vi "S30c_dll F101.vi"() -> ()   [LabVIEW 2014, in "K_S30c_dll.lvlib"]
uses:
  K_S30c_dll.lvlib
  s30c.dll
panel:
  in  "Parameter 0 .. 5":u8[](array[numeric])
  out "Org. Parameter 0 .. 4":u8[](array[numeric])
  in  "Index":u8
  out "error out":errorcluster
  in  "error in":errorcluster
  in  "Dev Addr":u8=250
  # "Function101: Write a single configurtion byte, using funtion 100\n\nWarning!\n\nPlease be careful, using this function! \nWrong configuration changes the function of the device! \nMake sure that you save first the origignal configuration with function 100.\nIf your device supports F32 (5.20-4.1 and earlier), then use F33 instead of this function.\n\nusing s30c.dll\nKeller AG für Druckmesstechnik, 29.5.08 b.v."
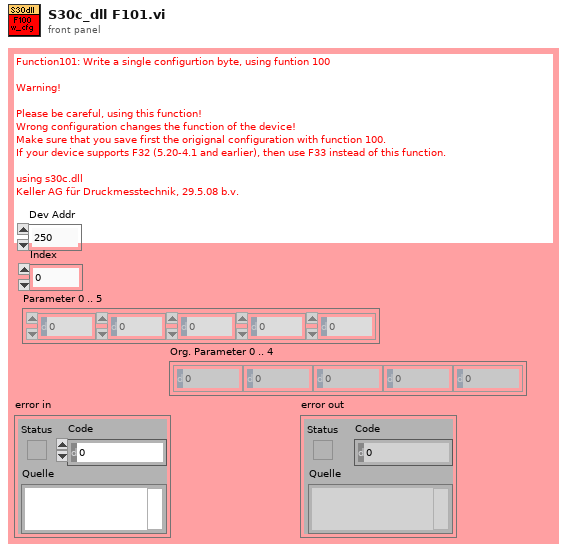
[diagram p1: front panel]
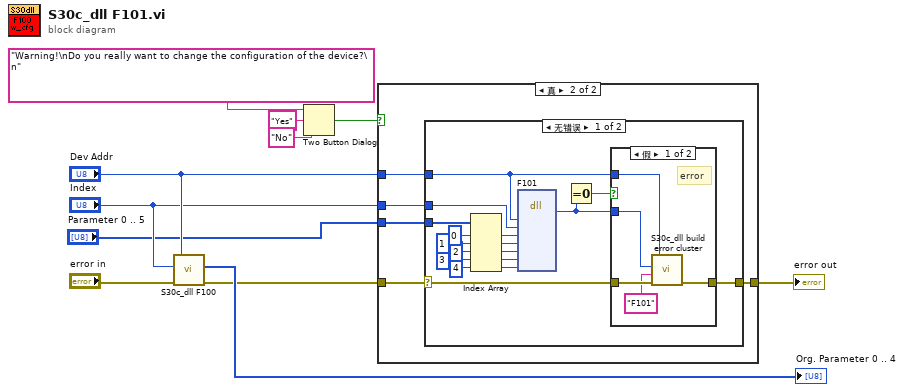
[diagram p0: block diagram]
diagram:
  n1 = call "S30c_dll F100.vi"("error in"="error in", "Index"="Index", "Dev Addr"="Dev Addr") -> ("error out"=w4:errorcluster, "Parameters 0 .. 4"=→"Org. Parameter 0 .. 4":u8[])  [unwired: 2 in, 1 out]
  n2 = Two Button Dialog(message="Warning!\nDo you really want to change the configuration of the device?\n" ("Nachricht"), 1:"No" ("F-Schaltflächenname (\"Abbrechen\")"), 2:"Yes" ("T-Schaltflächenname (\"OK\")")) -> (T button?=w3:bool)
  n3 = case shown="真" w3 {
    tunnel: [w12 w17] -> w8
    tunnel: "Dev Addr" -> [_ w16]
    tunnel: "Index" -> [_ w15]
    tunnel: w4 -> [w12 w14]
    tunnel: "Parameter 0 .. 5" -> [_ w13]
    frame False {
    }
    frame True {
      n4 = case shown="无错误" w14 {
        selector: w14 -> [w32 w41]
        tunnel: [w33 w41] -> w17
        tunnel: w16 -> [w23 _]
        tunnel: w15 -> [w24 _]
        tunnel: w13 -> [w25 _]
        frame No Error {
          n5 = Index Array(array=w25, index #1=0 ("Index"), index #2=1 ("Index"), index #3=2 ("Index"), index #4=3 ("Index"), index #5=4 ("Index")) -> (element #1=w26:u8, element #2=w27:u8, element #3=w28:u8, element #4=w29:u8, element #5=w30:u8)
          n6 = dll-call lib="PTH2Labs EworkSINOPEC北控自动相渗software2.08.5_dlls30c.dll" fn="F101"("DevAddr"=w23, "index"=w24, "Para0"=w26, "Para1"=w27, "Para2"=w28, "Para3"=w29, "para4"=w30) -> (w31:i16)  [unwired: 10 in, 2 out]
          n7 = Equal To 0?(x=w31) -> (x = 0?=w34:bool)
          n8 = case shown="假" w34 {
            tunnel: w32 -> [w39 w40]
            tunnel: [w38 w40] -> w33
            tunnel: w23 -> [w36 _]
            tunnel: w31 -> [w35 _]
            frame False {
              # "error"
              n9 = call "S30c_dll build error cluster.vi"("error in"=w39, "error Text"="F101", "error code"=w35, "Dev Addr"=w36) -> ("error out"=w38:errorcluster)  [unwired: 3 in]
            }
            frame True {
            }
          }
        }
        frame Error {
        }
      }
    }
  }
  "error out" <- w8
